vi "Read.vi"(8 "error in (no error)":errorcluster, 11 "Instrument Interface in":refnum<class "Instrument.lvclass">) -> (0 "error out":errorcluster, 2 "Data":string, 3 "Instrument Interface out":refnum<class "Instrument.lvclass">)   [LabVIEW 2020, in "Low Level PSU With Tests.lvlib" / "Instrument.lvclass"]
uses:
  Instrument.lvclass
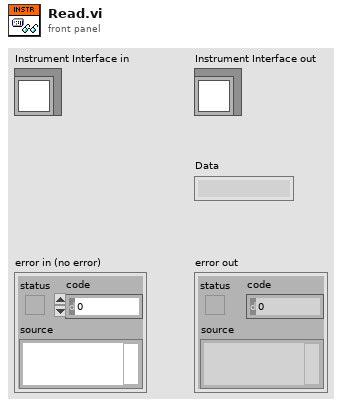
[diagram p1: front panel]
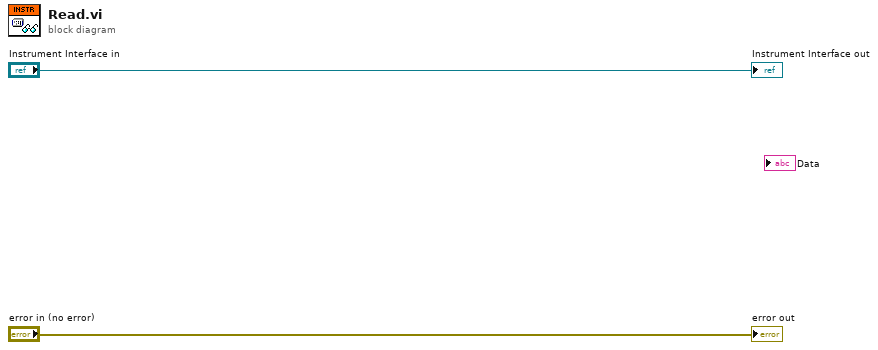
[diagram p0: block diagram]
diagram:
  "error out" <- "error in (no error)"
  "Instrument Interface out" <- "Instrument Interface in"
